vi "PicoScopeospaUnitInfo.vi"(7 "Mode":u16(ring) items=["Dialog On Error", "no dialog - CloseUnit and Stop", "no dialog - Continue", "no dialog - Stop"], 8 "error in (no error)":errorcluster, 11 "handle in":i16) -> (0 "error out":errorcluster, 2 "Unit Info":T1, 3 "handle out":i16)   [LabVIEW 2024]
doc: "Returns Driver and Unit Information"
uses:
  <vilib>/Utility/error.llb/Trim Whitespace One-Sided.vi
  psospa.dll
panel:
  out "json string":string
  out "outputStringLength":i32
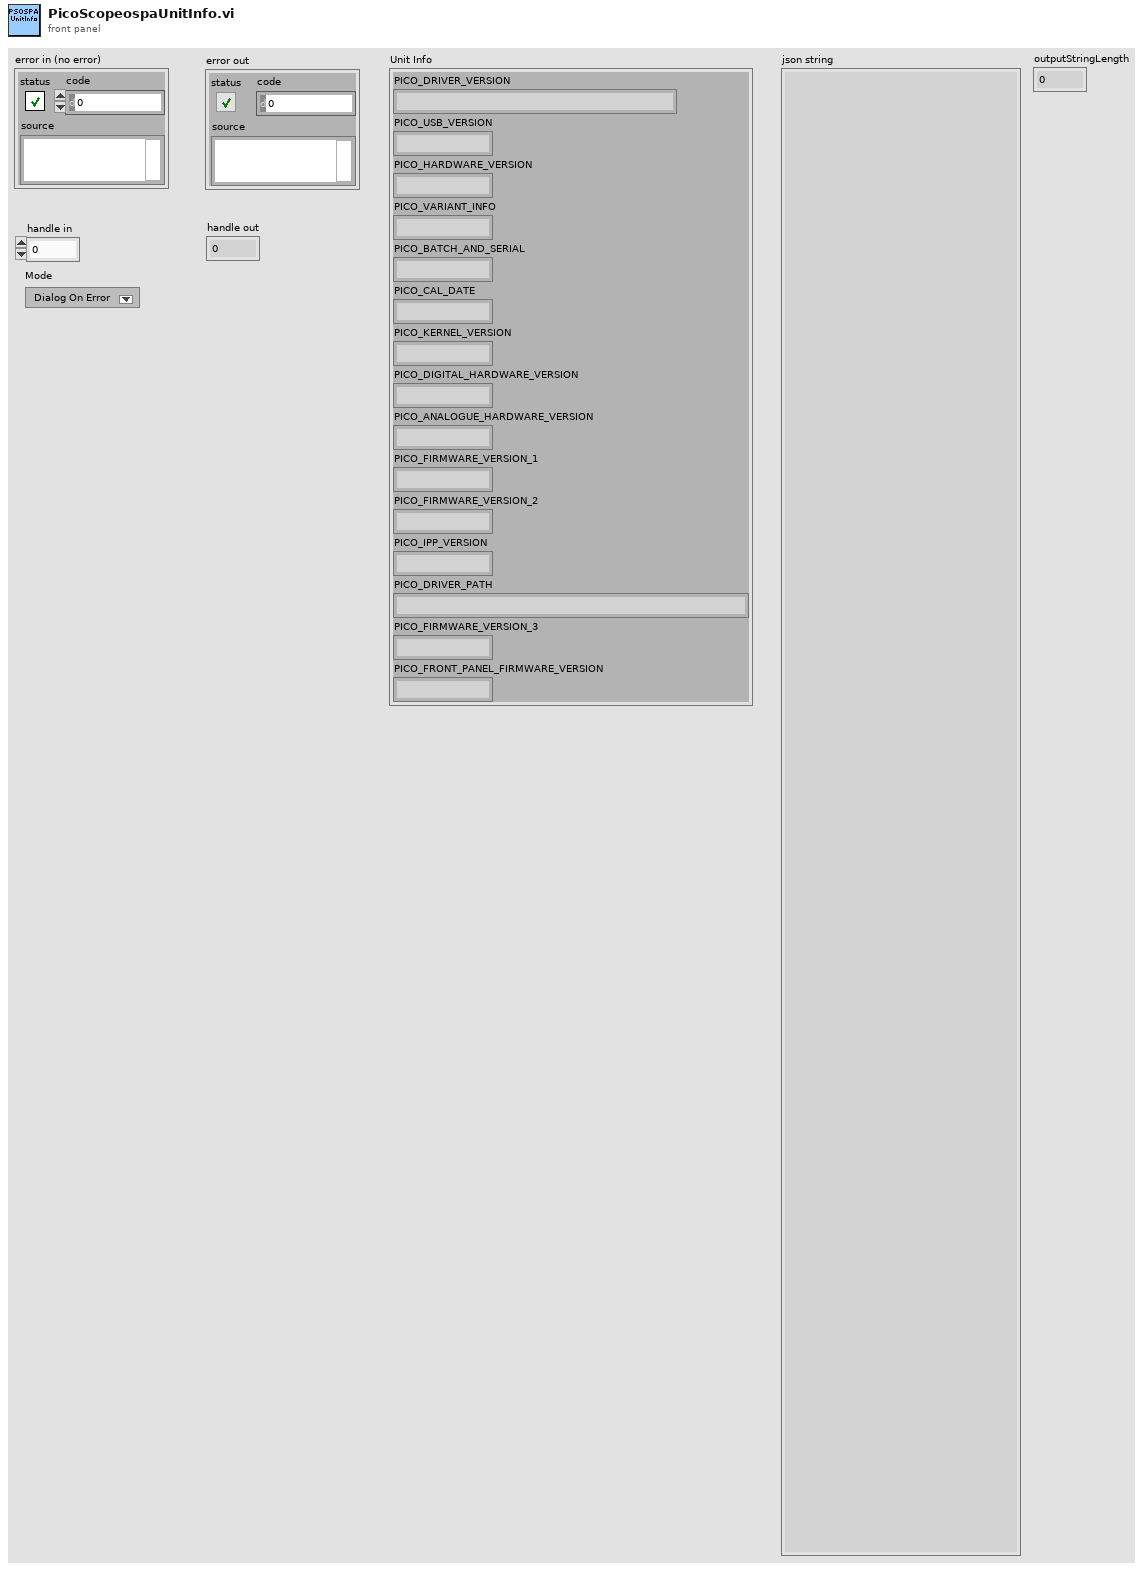
[diagram p1: front panel]
types:
  T1 = cluster{"PICO_DRIVER_VERSION":string, "PICO_USB_VERSION":string, "PICO_HARDWARE_VERSION":string, "PICO_VARIANT_INFO":string, "PICO_BATCH_AND_SERIAL":string, "PICO_CAL_DATE":string, "PICO_KERNEL_VERSION":string, "PICO_DIGITAL_HARDWARE_VERSION":string, "PICO_ANALOGUE_HARDWARE_VERSION":string, "PICO_FIRMWARE_VERSION_1":string, "PICO_FIRMWARE_VERSION_2":string, "PICO_IPP_VERSION":string, "PICO_DRIVER_PATH":string, "PICO_FIRMWARE_VERSION_3":string, "PICO_FRONT_PANEL_FIRMWARE_VERSION":string}
  T2 = cluster{"status":bool, "code":u32, "source":string}
  T3 = cluster{"[0]":string, "[1]":string, "[2]":string, "[3]":string, "[4]":string, "[5]":string, "[6]":string, "[7]":string, "[8]":string, "[9]":string, "[10]":string, "[11]":string, "[12]":string, "[13]":string, "[14]":string}
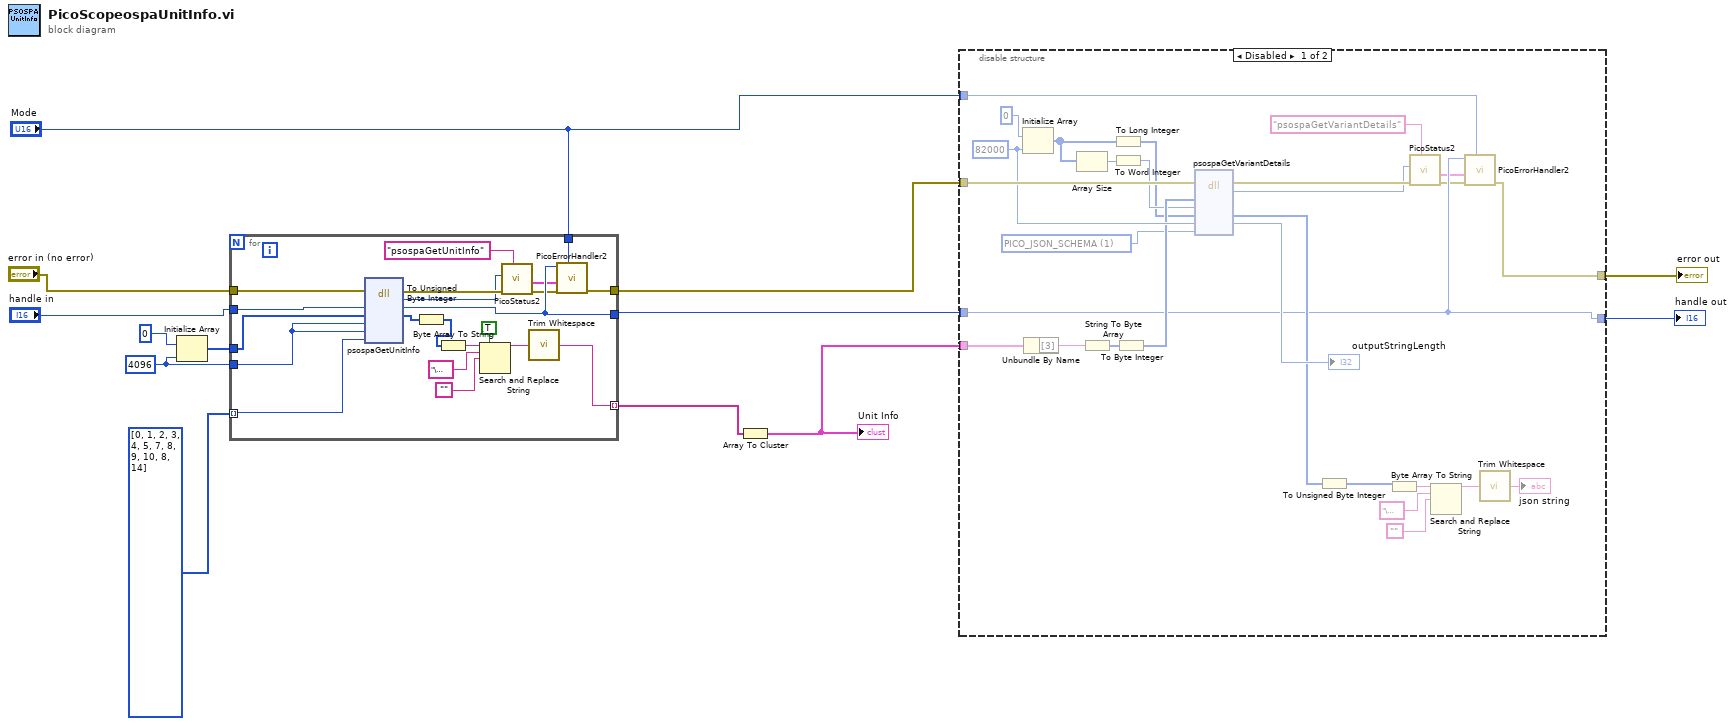
[diagram p0: block diagram]
diagram:
  w3 = i16 4096 ("requiredSize")
  n1 = Initialize Array(i8 0 ("element"), w3) -> (w5:i8[])
  n2 = for {
    tunnel: "error in (no error)" -> [w28]
    tunnel: [w20] -> w10
    tunnel: w5 -> [w29]
    tunnel: "handle in" -> [w27]
    tunnel: w3 -> [w26]
    tunnel: [w22] -> w8
    tunnel: u32[] [0, 1, 2, 3, 4, 5, 7, 8, 9, 10, 8, 14] ("initialized array") -> [w23] mode=indexing
    tunnel: [w21] -> w2 mode=indexing
    tunnel: "Mode" -> [w14]
    n3 = dll-call lib="F:/Picoscope3000e/Scope_LabView/ps3000e/Treiber_und_SubVis/psospa.dll" fn="psospaGetUnitInfo"(error in=w28, "handle"=w27, "string"=w29, "stringLength"=w26, "requiredSize"=w26, "deviceInfo"=w23) -> (error out=w16:errorcluster, "PICO_STATUS"=w15:u32, "handle"=w22:i16, "string"=w25:i8[])  [unwired: 5 in, 1 out]
    n4 = To Unsigned Byte Integer(number=w25) -> (unsigned 8bit integer=w24:u8[])
    n5 = Byte Array To String(unsigned byte array=w24) -> (string=w33:string)
    n6 = Search and Replace String(replace all?=TRUE ("replace all? (F)"), input string=w33, search string="\u0000", replace string="") -> (result string=w32:string)  [unwired: 4 in, 3 out]
    n7 = call "PicoStatus2.vi"("PICO source"="psospaGetUnitInfo" ("source"), "Error in"=w16, "PICO STATUS"=w15) -> ("error out"=w19:errorcluster, "PICO_STATUS out"=w18:T2)  [unwired: 5 in]
    n8 = call <vilib>:"Trim Whitespace.vi"("string"=w32) -> ("trimmed string"=w21:string)  [unwired: 1 in]
    n9 = call "PicoErrorHandler2.vi"("Mode"=w14, "error in (no error)"=w19, "PICO_STATUS in"=w18, "handle In"=w22) -> ("error out"=w20:errorcluster)  [unwired: 7 in]
  }
  n10 = Array To Cluster(array=w2) -> (cluster=w9:T3)
  "Unit Info" <- w9
  n11 = disable-structure shown="Disabled" {
    disable-tunnel: [w62 w63] -> w11
    disable-tunnel: w10 -> [w61 w63]
    disable-tunnel: w9 -> [w58 _]
    disable-tunnel: w8 -> [w41 w64]
    disable-tunnel: [w41 w64] -> w7
    disable-tunnel: "Mode" -> [w35 _]
    frame Disabled {
      w42 = u32 1 items=["PICO_JSON_DATA", "PICO_JSON_SCHEMA"] ("PICO_TEXT_FORMAT")
      w59 = 82000 ("dimension size")
      n12 = Initialize Array(i8 0 ("element"), w59) -> (w44:i8[])
      n13 = Unbundle By Name(w58) -> ("[3]"=w57:string)
      n14 = Array Size(array=w44) -> (size(s)=w45:i32)
      n15 = String To Byte Array(string=w57) -> (unsigned byte array=w56:u8[])
      n16 = To Long Integer(number=w44) -> (32bit integer=w43:i32[])
      n17 = To Word Integer(number=w45) -> (16bit integer=w46:i16)
      n18 = To Byte Integer(number=w56) -> (8bit integer=w55:i8[])
      n19 = dll-call lib="F:/Picoscope3000e/Scope_LabView/ps3000e/Treiber_und_SubVis/psospa.dll" fn="psospaGetVariantDetails"(error in=w61, "variantName"=w55, "variantNameLength"=w46, "outputString"=w43, "outputStringLength"=w59, "textFormat"=w42) -> (error out=w39:errorcluster, "PICO_STATUS"=w37:u32, "outputString"=w48:i32[], "outputStringLength"=→"outputStringLength":i32)  [unwired: 5 in, 1 out]
      n20 = To Unsigned Byte Integer(number=w48) -> (unsigned 8bit integer=w49:u8[])
      n21 = Byte Array To String(unsigned byte array=w49) -> (string=w52:string)
      n22 = call "PicoStatus2.vi"("PICO source"="psospaGetVariantDetails" ("source"), "Error in"=w39, "PICO STATUS"=w37) -> ("error out"=w40:errorcluster, "PICO_STATUS out"=w36:T2)  [unwired: 5 in]
      n23 = Search and Replace String(input string=w52, search string="\u0000", replace string="") -> (result string=w51:string)  [unwired: 5 in, 3 out]
      n24 = call "PicoErrorHandler2.vi"("Mode"=w35, "error in (no error)"=w40, "PICO_STATUS in"=w36, "handle In"=w41) -> ("error out"=w62:errorcluster)  [unwired: 7 in]
      n25 = call <vilib>:"Trim Whitespace.vi"("string"=w51) -> ("trimmed string"=→"json string":string)  [unwired: 1 in]
    }
    frame Enabled {
    }
  }
  "error out" <- w11
  "handle out" <- w7
